vi "new FGGA_10Hz_test.vi"(0 "VISA resource name out":refnum<visa-resource-name>, 11 "error IO":errorcluster) -> ()   [LabVIEW 2014]
uses:
  <vilib>/Instr/_visa.llb/VISA Set IO Buffer Mask.ctl
  <vilib>/Instr/_visa.llb/VISA Flush IO Buffer Mask.ctl
  <vilib>/Instr/_visa.llb/VISA Configure Serial Port (Instr).vi
  <vilib>/platform/TimedLoop/XDataNode/XDataNode.xnode
  <vilib>/Platform/TimedLoop/XDataNode/nitl_modes.ctl
  <vilib>/Platform/TimedLoop/XDataNode/XDNodeRunTimeDep.lvlib
  <vilib>/Platform/TimedLoop/XDataNode/wakeup.ctl
  <vilib>/Platform/TimedLoop/XDataNode/timing_clust.ctl
panel:
  out "Waveform Chart 3":u32(graph)
  out "Max time diff":u32
  out "Max time diff":u32
  out "time diff":u32(graph)
  out "Loop count 2":i32
  out "Number of times \nRead time out 2":u32
  out "RAW DATA 2":string
  out "length 2":i32
  out "Waveform Chart 2":i32(graph)
  out "Waveform Chart":i32(graph)
  out "length":i32
  out "Serial error out":errorcluster
  out "RAW DATA":string
  in  "stop":bool
  out "Number of times \nRead time out":u32
  out "Loop count":i32
  # "Date"
  # "Time"
  # "CH4_wet_ppm"
  # "1"
  # "CO4_wet_ppm_sd"
  # "H2O_ppm"
  # "3"
  # "H2O_ppm_sd"
  # "CO2_wet_ppm"
  # "5"
  # "CO2_wet_ppm_sd"
  # "CH4_dry_ppm"
  # "CH4_dry_ppm_sd"
  # "CO2_dry_ppm"
  # "CO2_dry_ppm_sd"
  # "cell_pressure_torr"
  # "11"
  # "cell_pressure_torr_sd"
  # "13"
  # "cell_temp_degC"
  # "cell_temp_degC_sdev"
  # "ambient(bench)_temp_degC"
  # "15"
  # "ambient(bench)_temp_dedgC_sd"
  # "17"
  # "RDA_us"
  # "RDA_us_sd"
  # "RDB_us"
  # "19"
  # "RDB_us_sd"
  # "Fitflag"
  # "21"
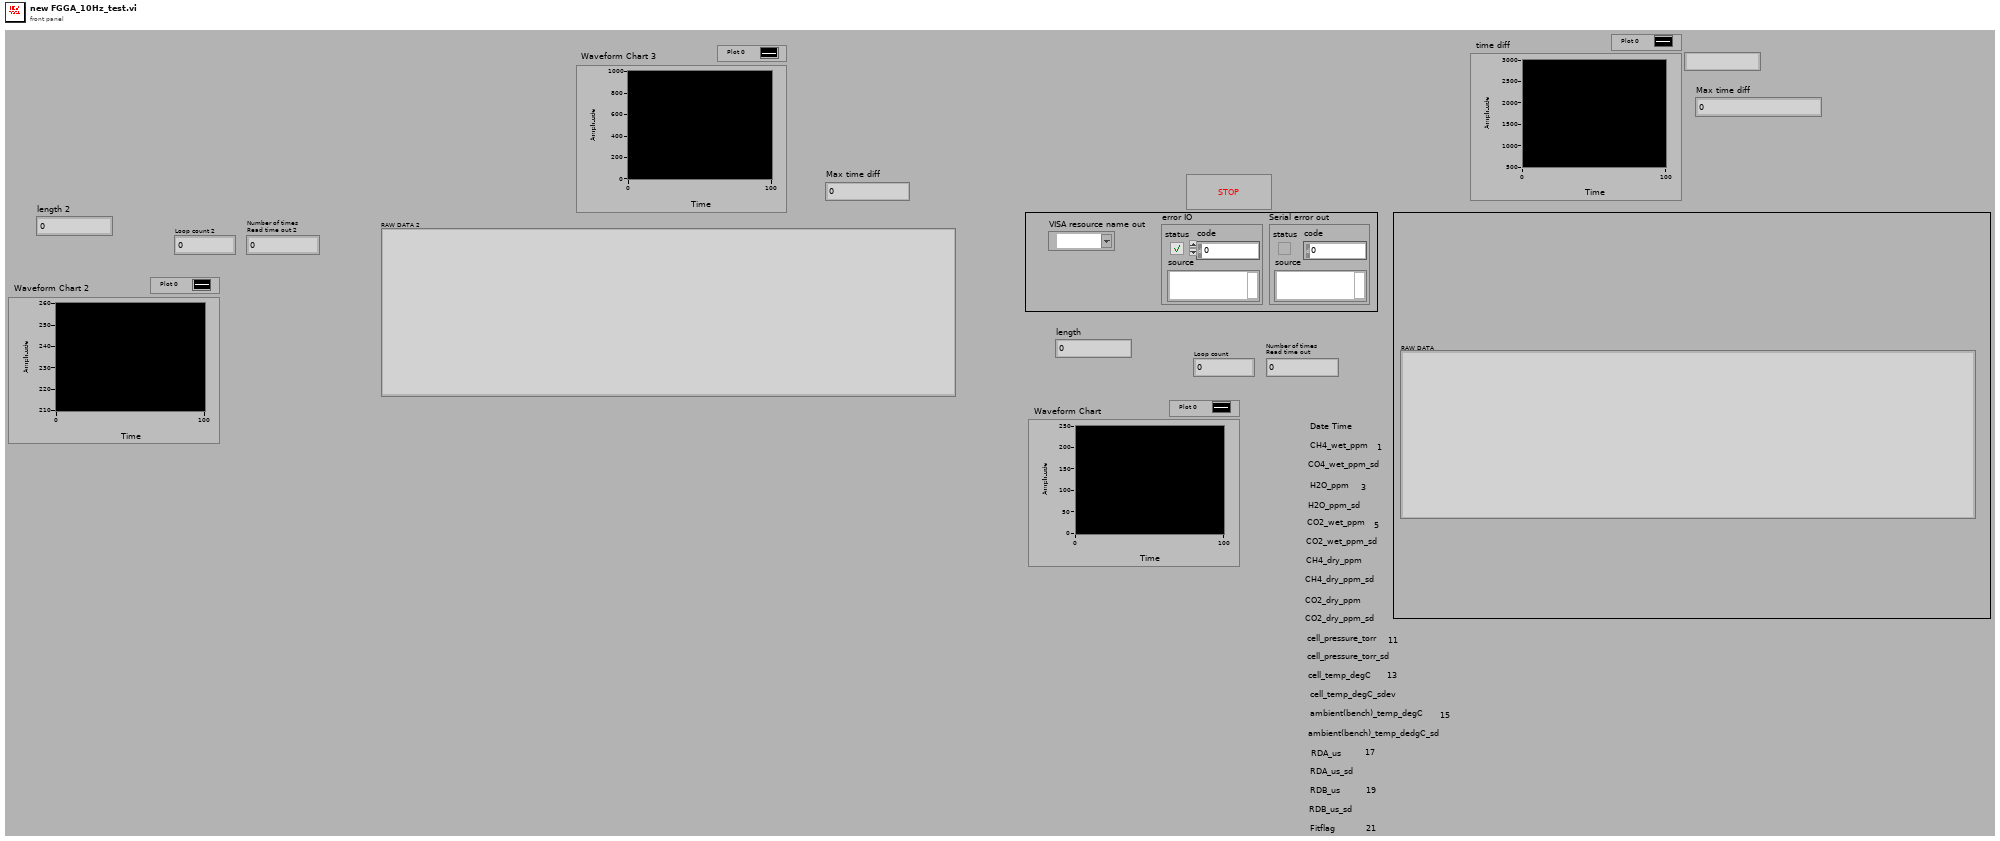
[diagram p1: front panel]
types:
  T1 = typedef "VISA Flush IO Buffer Mask.ctl" = u16
  T2 = typedef "VISA Set IO Buffer Mask.ctl" = u16
  T3 = typedef "XDNodeRunTimeDep.lvlib/timing_clust.ctl" = cluster{"Expected End [f-1]":u64, "Actual End [f-1]":u64, "Finished Late? [f-1]":bool, "Expected End [i-1]":u64, "Actual End [i-1]":u64, "Finished Late? [i-1]":bool, "Expected Start [i]":u64, "Actual Start [i]":u64, "Expected Start [f]":u64, "Actual Start [f]":u64, "Source Name":string, "Structure Name":string, "Period":i64, "Deadline":i64, "Offset":i64, "Start":i64, "Priority":i32, "Timeout":i32, "Mode":T4, "Wakeup Reason":T5, "Error":errorcluster, "Source Type":string, "Secondary Source Type":string, "Global End Time":u64, "Global Start Time":u64, "Frame Duration":u64, "Iteration Duration":u64, "Assigned CPU":i32, "I/O Scan Engine Mode":u32}
  T4 = typedef "XDNodeRunTimeDep.lvlib/nitl_modes.ctl" = enum32{"No Change", "Process missed periods, maintain original phase", "Discard missed periods, maintain original phase", "Process missed periods, ignore original phase", "Discard missed periods, ignore original phase"}
  T5 = typedef "XDNodeRunTimeDep.lvlib/wakeup.ctl" = enum32{"Normal", "Aborted", "Asynchronous wakeup", "Timing source error", "Timed loop error", "Timeout"}
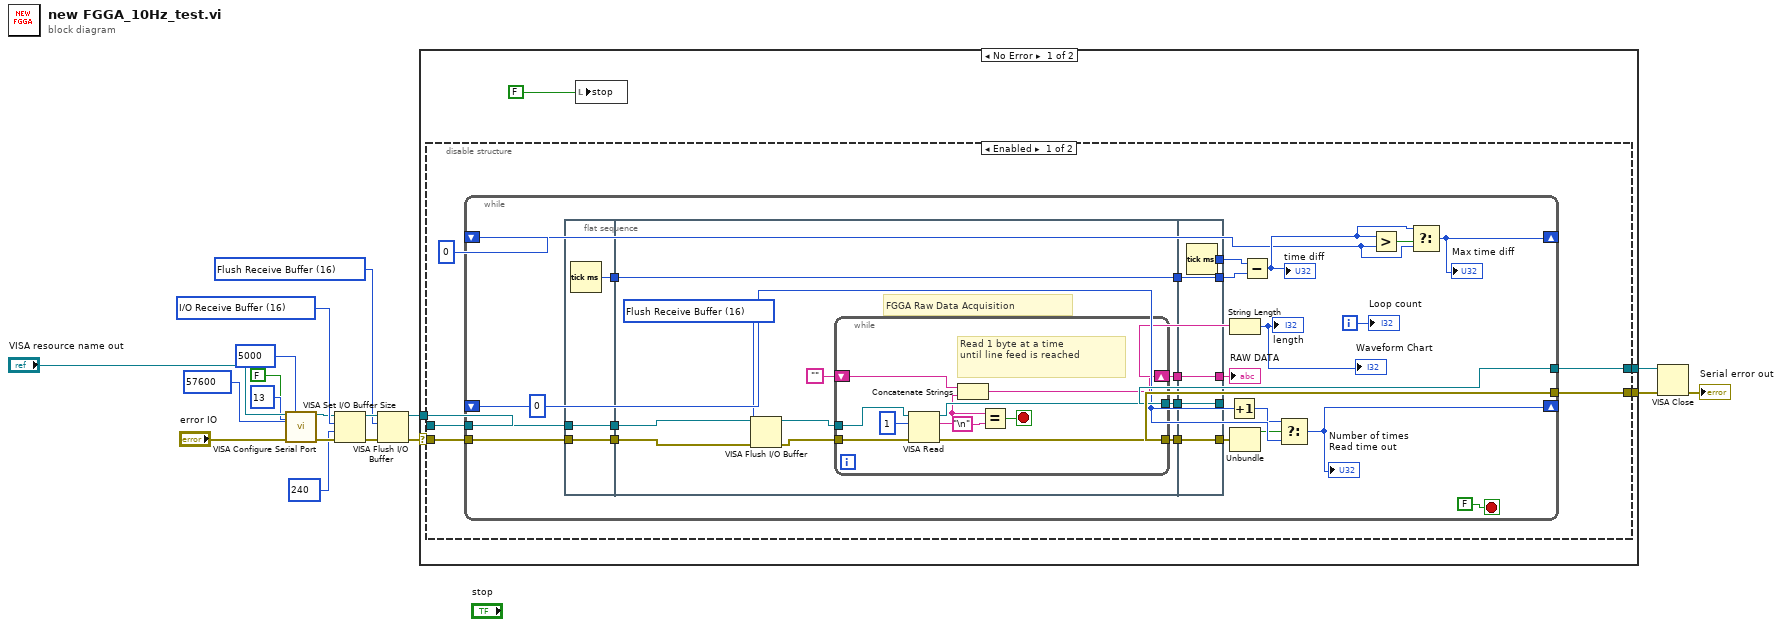
[diagram p0: block diagram]
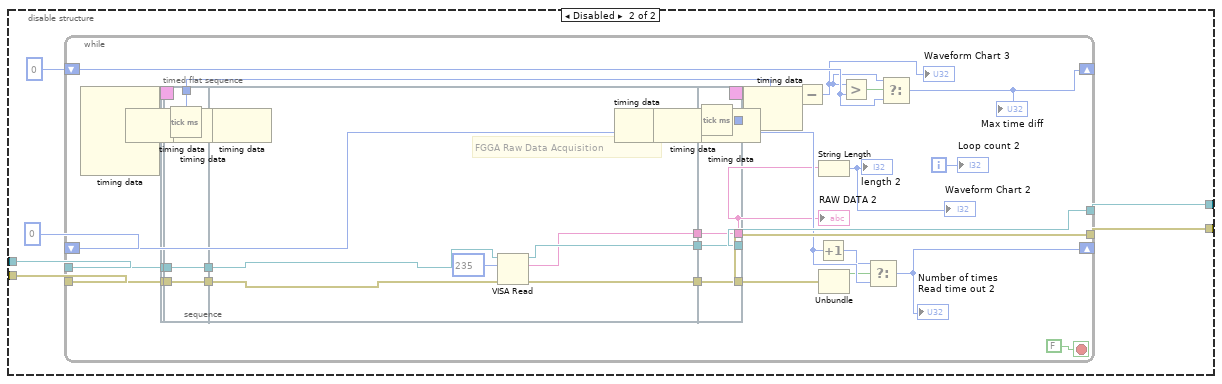
[diagram p2: hidden frame]
diagram:
  w9 = T1 16 items=["Flush Receive Buffer"=16, "Write Transmit Buffer to Device"=32, "Flush Receive Buffer (No I/O)"=64, "Flush Transmit Buffer"=128] ("Mask")
  w10 = T2 16 items=["I/O Receive Buffer"=16, "I/O Transmit Buffer"=32, "I/O Receive and Transmit Buffer"=48] ("Mask")
  n1 = call-poly "VISA Configure Serial Port"("VISA resource name"="VISA resource name out", "timeout (10sec)"=u32 5000, "termination char\n(0xA = '\\n' = LF)"=u8 13 ("termination char\n(0xA = '\\n' = LF)"), "Enable Termination\nChar (T)"=FALSE ("Enable Termination\nChar (T)"), "baud rate (9600)"=u32 57600, "error in (no error)"="error IO") -> ("VISA resource name out"=w8:refnum<visa-resource-name>, "error out"=w7:errorcluster)  [unwired: 8 in]
  n2 = VISA Set I/O Buffer Size(VISA resource name=w8, mask (16)=w10, size (4096)=u32 240, error in (no error)=w7) -> (VISA resource name out=w11:refnum<visa-resource-name>, error out=w12:errorcluster)
  n3 = VISA Flush I/O Buffer(VISA resource name=w11, mask (16)=w9, error in (no error)=w12) -> (VISA resource name out=w4:refnum<visa-resource-name>, error out=w3:errorcluster)
  n4 = case shown="No Error" w3 {
    selector: w3 -> [w19 w142]
    tunnel: w4 -> [w20 w143]
    tunnel: [w22 w143] -> w15
    tunnel: [w23 w142] -> w16
    frame No Error {
      n5 = disable-structure shown="Enabled" {
        disable-tunnel: [w29 w87] -> w23
        disable-tunnel: [w28 w88] -> w22
        disable-tunnel: w20 -> [w27 w86]
        disable-tunnel: w19 -> [w26 w85]
        frame Enabled {
          n6 = while {
            tunnel: w27 -> [w44]
            tunnel: w26 -> [w43]
            tunnel: [w54] -> w29
            shift-right: [w50] -> _
            shift-left: u32 0 -> [w51]
            tunnel: [w53] -> w28
            shift-right: [w37] -> _
            shift-left: u32 0 -> [w38]
            i -> [w52]
            stop <- FALSE stop-if-true
            n7 = flat-sequence {
              tunnel: w43 -> [w56]
              tunnel: w44 -> [w57]
              tunnel: [w57] -> w31
              tunnel: [w56] -> w32
              tunnel: [w55] -> w30
              tunnel: w31 -> [w60]
              tunnel: w32 -> [w59]
              tunnel: [w67] -> w33
              tunnel: [w66] -> w34
              tunnel: [w64] -> w35
              tunnel: [w58] -> w36
              tunnel: w30 -> [w58]
              tunnel: [w80] -> w46
              tunnel: [w81] -> w53
              tunnel: [w82] -> w54
              tunnel: w33 -> [w82]
              tunnel: w34 -> [w81]
              tunnel: w35 -> [w80]
              tunnel: [w79] -> w42
              tunnel: [w78] -> w41
              tunnel: w36 -> [w78]
              frame #0 {
                n8 = Tick Count (ms)() -> (millisecond timer value=w55:u32)
              }
              frame #1 {
                w61 = T1 16 items=["Flush Receive Buffer"=16, "Write Transmit Buffer to Device"=32, "Flush Receive Buffer (No I/O)"=64, "Flush Transmit Buffer"=128] ("Mask")
                # "FGGA Raw Data Acquisition"
                n9 = VISA Flush I/O Buffer(VISA resource name=w60, mask (16)=w61, error in (no error)=w59) -> (VISA resource name out=w62:refnum<visa-resource-name>, error out=w63:errorcluster)
                n10 = while {
                  tunnel: [w77] -> w66
                  tunnel: [w76] -> w67
                  tunnel: w62 -> [w75]
                  tunnel: w63 -> [w74]
                  shift-right: [w72] -> w64
                  shift-left: "" -> [w73]
                  stop <- w69 stop-if-true
                  # "Read 1 byte at a time \nuntil line feed is reached"
                  n11 = VISA Read(VISA resource name=w75, byte count=u32 1, error in (no error)=w74) -> (VISA resource name out=w77:refnum<visa-resource-name>, read buffer=w71:string, error out=w76:errorcluster)  [unwired: 1 out]
                  n12 = Concatenate Strings(w73, w71) -> (w72:string)
                  n13 = Equal?(x=w71, y="\n") -> (x = y?=w69:bool)
                }
              }
              frame #2 {
                n14 = Tick Count (ms)() -> (millisecond timer value=w79:u32)
              }
            }
            n15 = Increment(x=w51) -> (x+1=w49:u32)
            n16 = String Length(string=w46) -> (length=→"length" →"Waveform Chart":i32)
            n17 = Unbundle(w54) -> ("status"=w48:bool)  [unwired: 2 out]
            n18 = Subtract(x=w42, y=w41) -> (x-y=w39:u32)
            "time diff" <- w39
            n19 = Select(t=w49, s=w48, f=w51) -> (s? t:f=w50:u32)
            "Number of times \nRead time out" <- w50
            n20 = Greater?(x=w39, y=w38) -> (0:w40:bool)
            n21 = Select(t=w39, s=w40, f=w38) -> (s? t:f=w37:u32)
            "Max time diff" <- w37
            "Loop count" <- w52
            "RAW DATA" <- w46
          }
        }
        frame Disabled {
          n22 = while {
            tunnel: w86 -> [w99]
            tunnel: w85 -> [w98]
            tunnel: [w108] -> w87
            shift-right: [w104] -> _
            shift-left: 0 -> [w105]
            tunnel: [w107] -> w88
            shift-right: [w92] -> _
            shift-left: u32 0 -> [w93]
            i -> [w106]
            stop <- FALSE stop-if-true
            n23 = node-c288() -> (w90:T3)  [unwired: 4 in]
            n24 = timed-sequence {
              timing: w90 -> [_]
              timing-out: [_] -> w89
              tunnel: w99 -> [w120]
              tunnel: w98 -> [w119]
              tunnel: [w118] -> w95
              tunnel: [w114] -> w108
              tunnel: [w112] -> w107
              tunnel: [w110] -> w97
              tunnel: [w109] -> w96
              n25 = timed-flat-sequence {
                tunnel: w119 -> [w122]
                tunnel: w120 -> [w123]
                tunnel: [w123] -> w117
                tunnel: [w122] -> w116
                tunnel: [w121] -> w118
                tunnel: [w131] -> w115
                tunnel: [w130] -> w113
                tunnel: [w128] -> w111
                tunnel: w117 -> [w127]
                tunnel: w116 -> [w126]
                tunnel: [w135] -> w110
                tunnel: [w136] -> w112
                tunnel: [w137] -> w114
                tunnel: w115 -> [w137]
                tunnel: w113 -> [w136]
                tunnel: w111 -> [w135]
                tunnel: [w134] -> w109
                frame #0 {
                  n26 = node-c288() -> ()  [unwired: 1 in, 1 out]
                  n27 = Tick Count (ms)() -> (millisecond timer value=w121:u32)
                  n28 = node-c288() -> ()  [unwired: 1 in, 1 out]
                }
                frame #1 {
                  # "FGGA Raw Data Acquisition"
                  n29 = node-c288() -> ()  [unwired: 1 in, 1 out]
                  n30 = VISA Read(VISA resource name=w127, byte count=u32 235, error in (no error)=w126) -> (VISA resource name out=w130:refnum<visa-resource-name>, read buffer=w128:string, error out=w131:errorcluster)  [unwired: 1 out]
                  n31 = node-c288() -> ()  [unwired: 1 in, 1 out]
                }
                frame #2 {
                  n32 = node-c288() -> ()  [unwired: 1 in, 1 out]
                  n33 = Tick Count (ms)() -> (millisecond timer value=w134:u32)
                  n34 = node-c288() -> ()  [unwired: 1 in, 1 out]
                }
              }
            }
            "RAW DATA 2" <- w97
            n35 = node-c288(w89) -> ()  [unwired: 1 out]
            n36 = Subtract(x=w96, y=w95) -> (x-y=w91:u32)
            "Waveform Chart 3" <- w91
            n37 = Increment(x=w105) -> (x+1=w103:i32)
            n38 = String Length(string=w97) -> (length=→"length 2" →"Waveform Chart 2":i32)
            n39 = Unbundle(w108) -> ("status"=w102:bool)  [unwired: 2 out]
            n40 = Greater?(x=w91, y=w93) -> (0:w94:bool)
            n41 = Select(t=w103, s=w102, f=w105) -> (s? t:f=w104:i32)
            "Number of times \nRead time out 2" <- w104
            n42 = Select(t=w91, s=w94, f=w93) -> (s? t:f=w92:u32)
            "Max time diff" <- w92
            "Loop count 2" <- w106
          }
        }
      }
      n43 = local write "stop"(FALSE ("stop")) -> ()
    }
    frame Error {
    }
  }
  n44 = VISA Close(VISA resource name=w15, error in (no error)=w16) -> (error out=→"Serial error out":errorcluster)
